vi "ConnectDSA.vi"(3 "error in (no error)":errorcluster, 4 "timeout ms (20000)":i32=20000, 5 "address":string) -> (0 "error out":errorcluster, 1 "connection ID out":refnum<k5>)   [LabVIEW 2015]
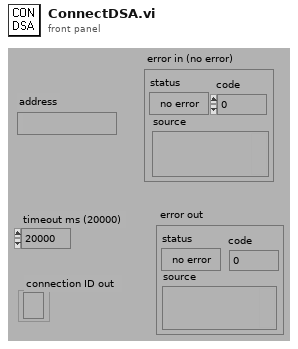
[diagram p1: front panel]
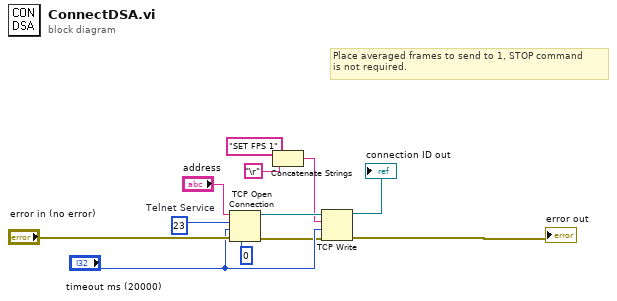
[diagram p0: block diagram]
diagram:
  w5 = 23  # Telnet Service
  # "Place averaged frames to send to 1, STOP command\nis not required."
  n1 = TCP Open Connection(address="address", remote port or service name=w5, timeout ms (60000)="timeout ms (20000)", local port=u16 0, error in (no error)="error in (no error)") -> (connection ID=w9:refnum<k5>, error out=w10:errorcluster)
  n2 = Concatenate Strings("SET FPS 1", "\r") -> (w8:string)
  n3 = TCP Write(connection ID=w9, data in=w8, error in (no error)=w10, 9:"timeout ms (20000)") -> (connection ID out=→"connection ID out":refnum<k5>, error out=→"error out":errorcluster)  [unwired: 1 out]
